vi "Increase Coordinate Count (Keith Koch's conflicted copy 2013-05-10).vi"   [LabVIEW 2011]
uses:
  _GlobalVariables&Libraries/ATV Program Global Variables.vi
types:
  T1 = cluster{"Navigation Coordinates":cluster{"Latitude":dbl, "Longitude":dbl}[], "Coordinate Count":u32, "Drive Speed":string, "Steer Angle":dbl, "Steering":dbl, "Direction to next Coordinate":dbl, "Drive":dbl, "Navigation Path":string}
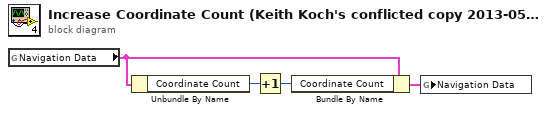
[diagram p0: block diagram]
diagram:
  n1 = global read "ATV Program Global Variables.vi" "Navigation Data"() -> (w4:T1)
  n2 = Unbundle By Name(w4) -> ("Coordinate Count"=w2:u32)
  n3 = Increment(x=w2) -> (x+1=w1:u32)
  n4 = Bundle By Name(cluster=w4, "Coordinate Count"=w1) -> (w3:T1)
  n5 = global write "ATV Program Global Variables.vi" "Navigation Data"(w3) -> ()
